vi "GetGlobalDefaultConfiguration.vi"(3 "Read defaults?":bool) -> ()   [LabVIEW 2013]
uses:
  QC_MeasurementSetup.vi
panel:
  out "Configuration File Striptest":path
  out "Configuration File Cis":path
  out "Configuration File Stability":path
  out "Configuration File CV":path
  out "Configuration File IV":path
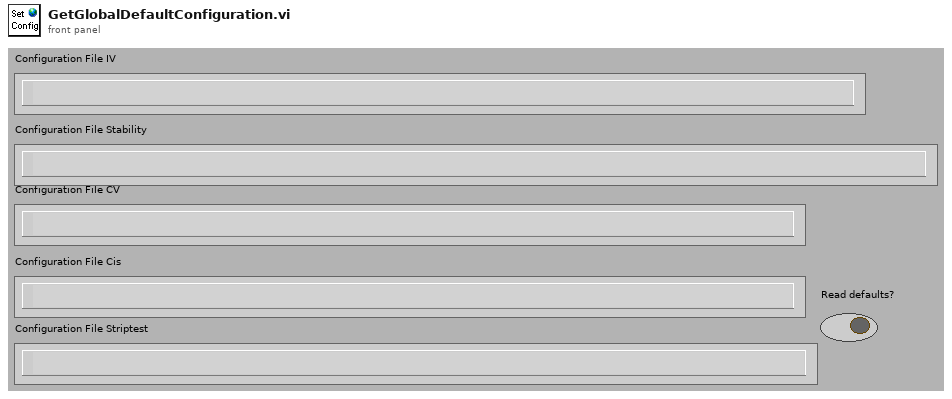
[diagram p1: front panel]
types:
  T1 = cluster{"Supply":refnum<class "SupplyControl.lvclass">, "Arduino":refnum<class "ArduinoControl.lvclass">, "Measurement switch":refnum<class "Switching.lvclass">, "Initial Voltage [V]":dbl, "Final Voltage [V]":dbl, "Step Size [V]":dbl, "Step Interval [s]":i32, "Number Of Steps":u32, "Ramp down steps [V]":dbl, "Ramp down Interval [s]":i32, "hold steps":i32, "Set Current Limit?":bool, "Current Limit [µA]":dbl, "Temperature Readout":enum16{"Read Arduino", "Enter manually"}, "Supply Name":string, "V_breakdown Limit [V]":dbl, "Measurement switch used?":bool}
  T2 = cluster{"Supply":refnum<class "SupplyControl.lvclass">, "LCR":refnum<class "LCRControl.lvclass">, "Arduino":refnum<class "ArduinoControl.lvclass">, "Measurement switch":refnum<class "Switching.lvclass">, "Initial Voltage [V]":dbl, "Final Voltage [V]":dbl, "Step Size [V]":dbl, "Step Interval [s]":i32, "Number Of Steps":u32, "AC frequency [Hz]":i32, "RC Configuration":u16, "AC amplitude [V]":dbl, "Ramp down steps [V]":dbl, "Ramp down Interval [s]":i32, "Set Current Limit?":bool, "Current Limit [µA]":dbl, "Temperature Readout":enum16{"Read Arduino", "Enter manually"}, "Supply Name":string, "LCR Name":string, "V_depletion Limit [V]":dbl, "Measurement switch used?":bool}
  T3 = cluster{"Supply":refnum<class "SupplyControl.lvclass">, "DMM":refnum<class "MultimeterControl.lvclass">, "DUT switch":refnum<class "Switching.lvclass">, "Arduino":refnum<class "ArduinoControl.lvclass">, "Measurement switch":refnum<class "Switching.lvclass">, "Voltage [V]":dbl, "Measurement Interval [s]":i32, "Test Duration":u32, "Ramp up steps [V]":dbl, "Ramp up Interval [s]":u32, "Ramp down steps [V]":dbl, "Ramp down Interval [s]":i32, "Set Current Limit?":bool, "Current Limit [µA]":dbl, "Temperature Readout":enum16{"Read Arduino", "Enter manually"}, "Supply Name":string, "DMM Name":string, "Maximum current fluctuation [%]":dbl, "Measurement switch used?":bool, "DUT switch used?":bool}
  T4 = cluster{"Supply":refnum<class "SupplyControl.lvclass">, "LCR":refnum<class "LCRControl.lvclass">, "Arduino":refnum<class "ArduinoControl.lvclass">, "Measurement switch":refnum<class "Switching.lvclass">, "Initial Voltage [V]":dbl, "Final Voltage [V]":dbl, "Step Size [V]":dbl, "Step Interval [s]":i32, "Number Of Steps":u32, "AC frequency [Hz]":i32, "RC Configuration":u16, "AC amplitude [V]":dbl, "Ramp down steps [V]":dbl, "Ramp down Interval [s]":i32, "Set Current Limit?":bool, "Current Limit [µA]":dbl, "Temperature Readout":enum16{"Read Arduino", "Enter manually"}, "Supply Name":string, "LCR Name":string, "C_is Limit [pF/cm]":dbl, "Measurement switch used?":bool}
  T5 = cluster{"Bias Supply":refnum<class "SupplyControl.lvclass">, "SMU":refnum<class "SupplyControl.lvclass">, "LCR":refnum<class "LCRControl.lvclass">, "ProbeStation":refnum<class "ProbeStationControl.lvclass">, "Arduino":refnum<class "ArduinoControl.lvclass">, "Measurement switch":refnum<class "Switching.lvclass">, "Probe Card Channels":i32, "Bias Voltage [V]":dbl, "First strip":i32, "Last strip":i32, "Base Voltage [V]":dbl, "Base Ramp Step [V]":dbl, "Base Ramp Interval [ms]":u32, "High Voltage [V]":dbl, "High Ramp Step [V]":dbl, "High Ramp Interval [ms]":u32, "AC frequency [Hz]":i32, "AC amplitude [V]":dbl, "RC Configuration":u16, "Single Needle":bool, "Temperature Readout":enum16{"Read Arduino", "Enter manually"}, "Fraction of good strips [%]":dbl, "Measurement switch used?":bool, "Matrix X Channels":cluster{"Mux1 C1":i32, "Mux1 C2":i32, "Mux2 C1":i32, "Mux2 C2":i32}, "Pinholes Y/N":bool, "Capacitance Y/N":bool, "Resistance Y/N":bool, "Bias Supply Name":string, "SMU Name":string, "LCR Name":string}
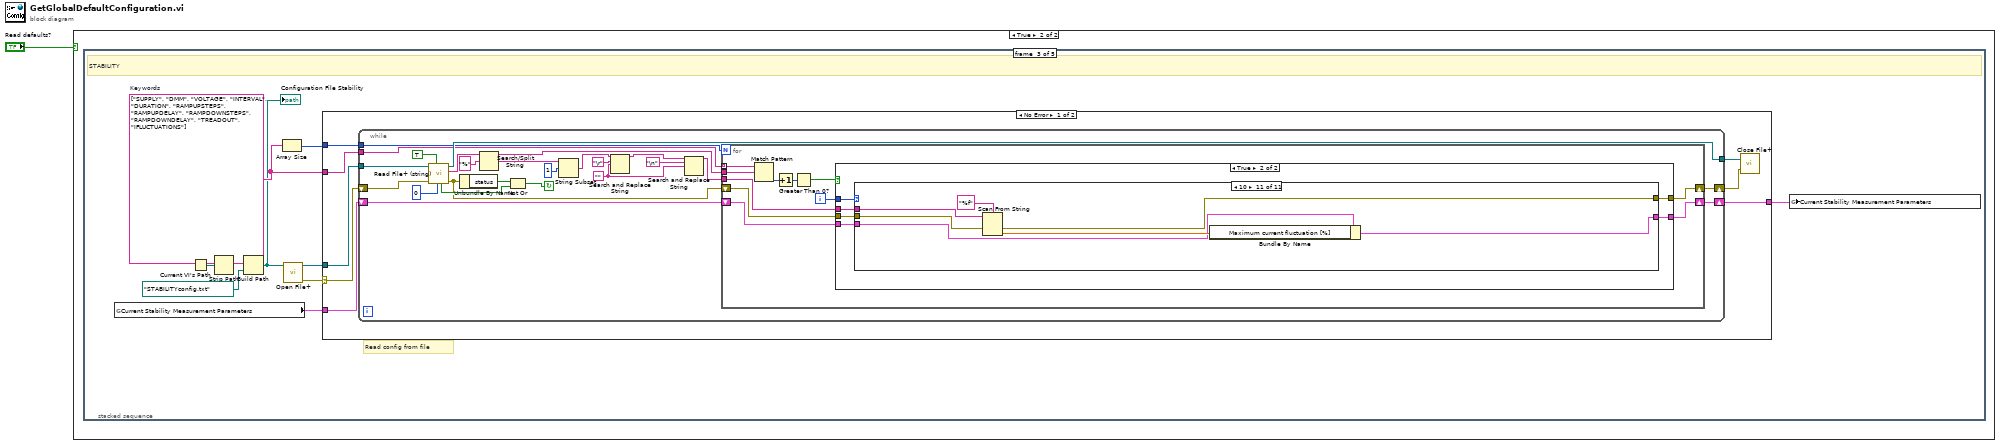
[diagram p0: block diagram]
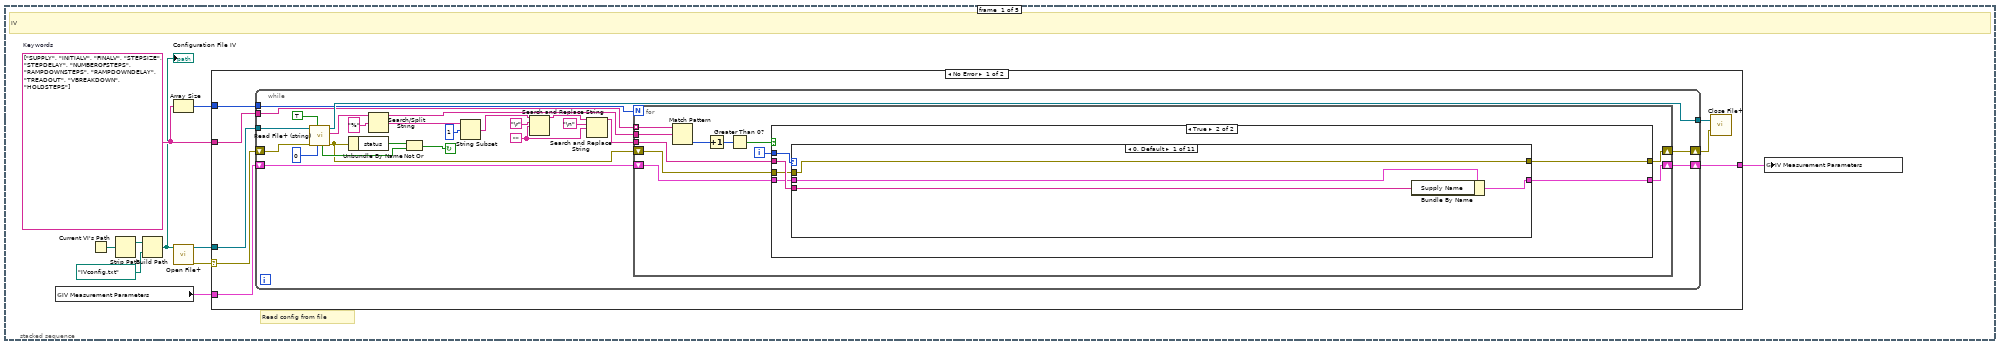
[diagram p3: hidden frame]
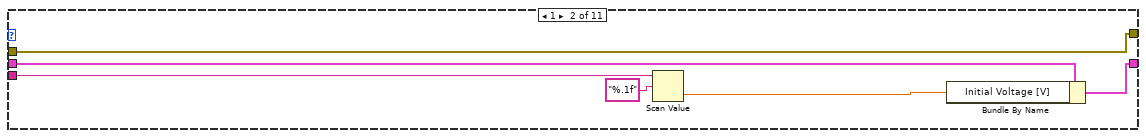
[diagram p5: hidden frame]
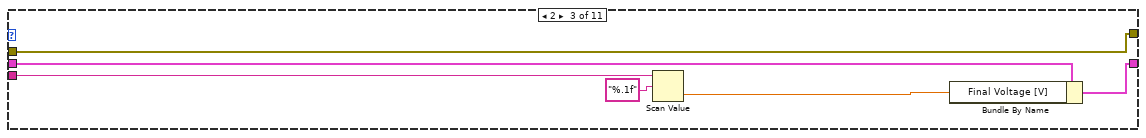
[diagram p6: hidden frame]
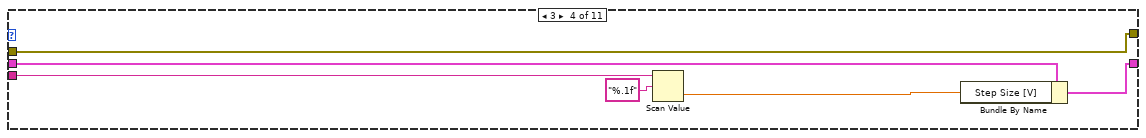
[diagram p7: hidden frame]
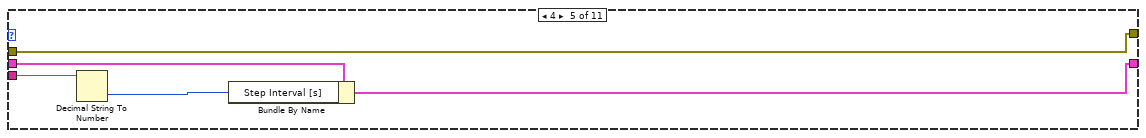
[diagram p8: hidden frame]
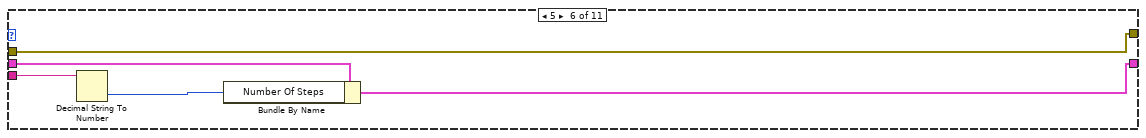
[diagram p9: hidden frame]
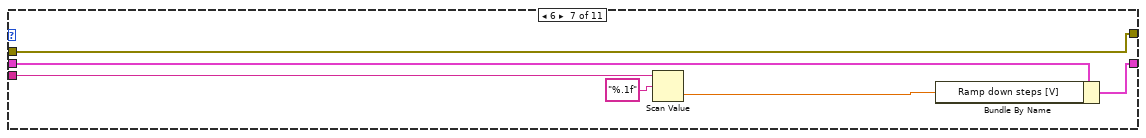
[diagram p10: hidden frame]
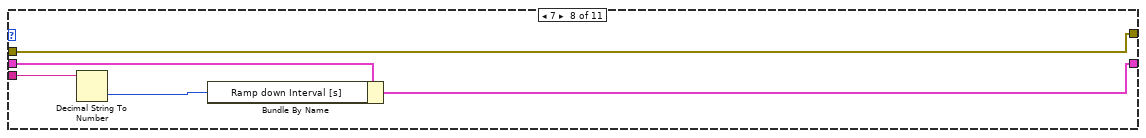
[diagram p11: hidden frame]
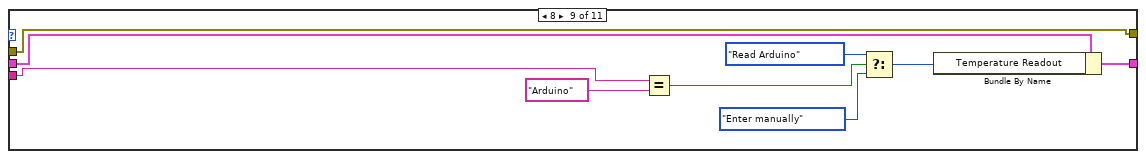
[diagram p12: hidden frame]
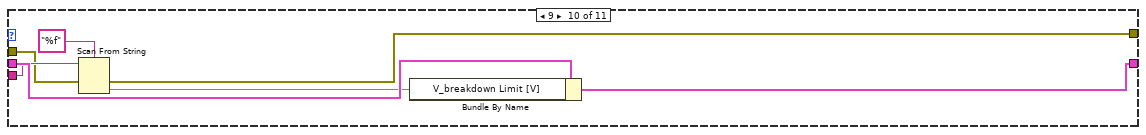
[diagram p13: hidden frame]
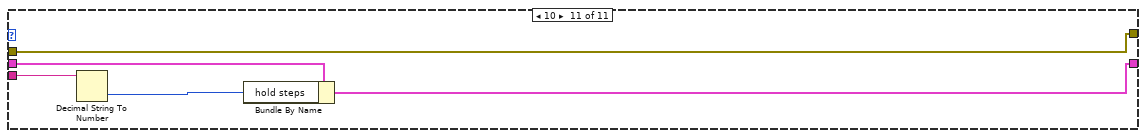
[diagram p14: hidden frame]
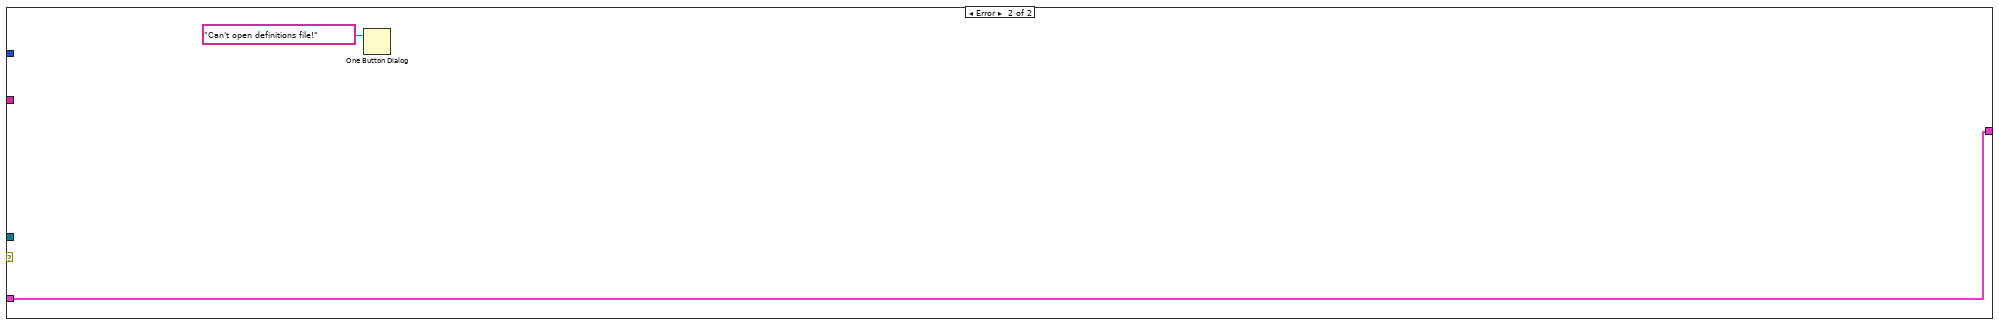
[diagram p15: hidden frame]
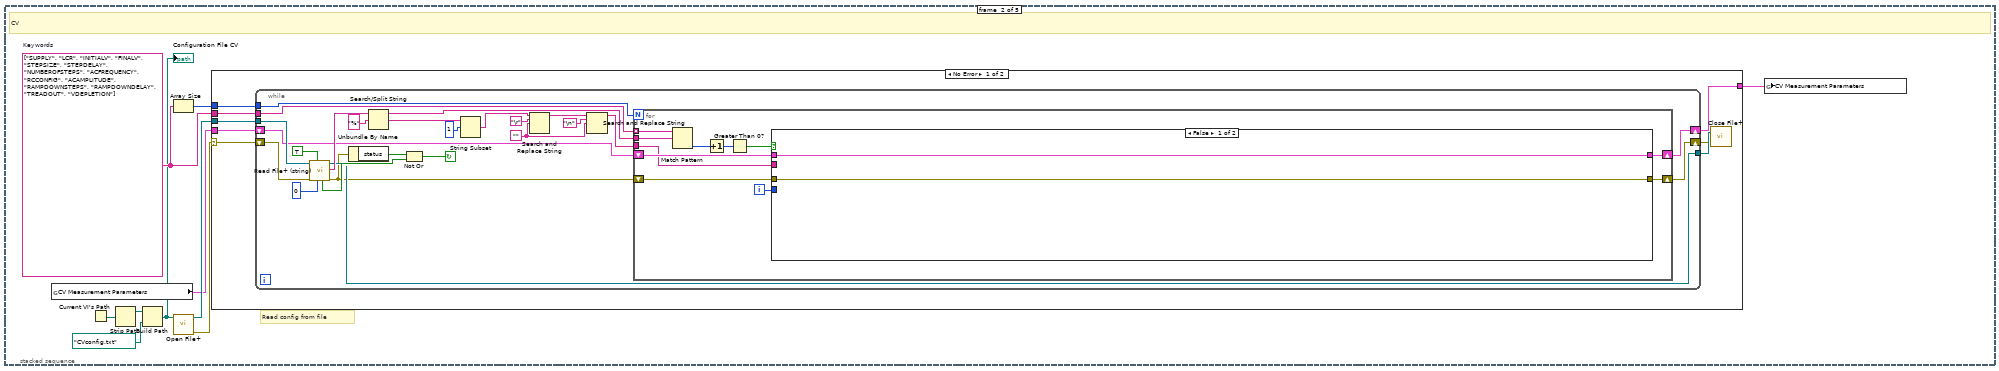
[diagram p16: hidden frame]
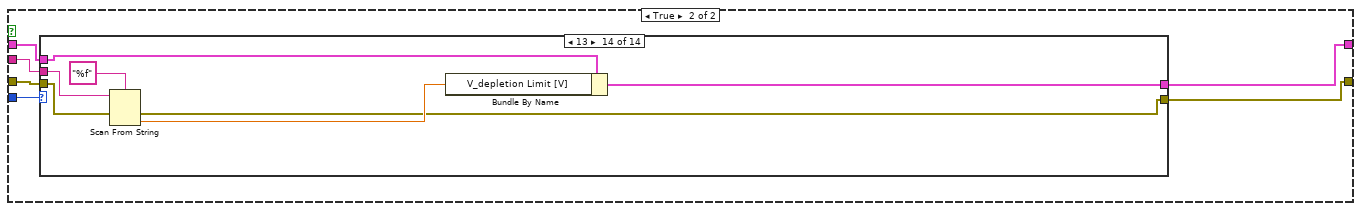
[diagram p17: hidden frame]
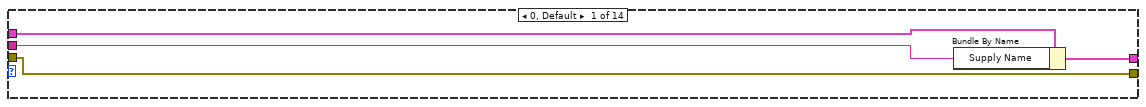
[diagram p18: hidden frame]
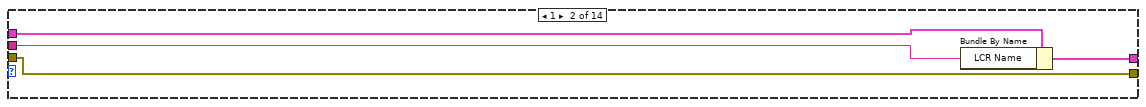
[diagram p19: hidden frame]
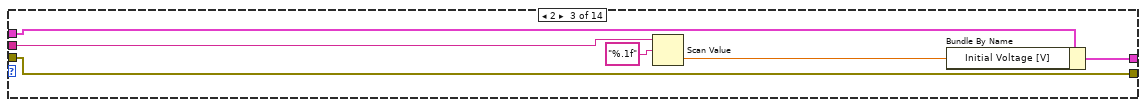
[diagram p20: hidden frame]
diagram:
  n1 = case shown="True" "Read defaults?" {
    frame False {
    }
    frame True {
      n2 = stacked-sequence {
        frame #0 {
          w11 = string[] ["SUPPLY", "INITIALV", "FINALV", "STEPSIZE", "STEPDELAY", "NUMBEROFSTEPS", "RAMPDOWNSTEPS", "RAMPDOWNDELAY", "TREADOUT", "VBREAKDOWN", "HOLDSTEPS"]  # Keywords
          # "Read config from file"
          # "IV"
          n3 = global read "QC_MeasurementSetup.vi" "IV Measurement Parameters"() -> (w2:T1)
          n4 = Current VI's Path() -> (path=w6:path)
          n5 = Strip Path(path=w6) -> (stripped path=w5:path)  [unwired: 1 out]
          n6 = Build Path(base path=w5, name or relative path=path "IVconfig.txt") -> (appended path=w4:path)
          "Configuration File IV" <- w4
          n7 = Array Size(array=w11) -> (size(s)=w10:i32)
          n8 = call <vilib>:"Open File+.vi"("file path (\" \")"=w4) -> ("error out"=w7:errorcluster, "refnum"=w8:refnum<file>)  [unwired: 7 in, 2 out]
          n9 = case shown="No Error" w7 {
            selector: w7 -> [w12 _]
            tunnel: w8 -> [w19 _]
            tunnel: w11 -> [w18 _]
            tunnel: w10 -> [w17 _]
            tunnel: w2 -> [w16 w128]
            tunnel: [w15 w128] -> w3
            frame No Error {
              n10 = while {
                shift-left: w16 -> [w30]
                shift-right: [w29] -> w15
                tunnel: w17 -> [w28]
                tunnel: w18 -> [w32]
                tunnel: [w35] -> w14
                tunnel: w19 -> [w41]
                shift-right: [w26] -> w13
                shift-left: w12 -> [w34]
                stop <- w37 continue-if-true
                w23 = ""
                n11 = call <vilib>:"Read File+ (string).vi"("count"=0, "line mode (characters:F)"=TRUE, "error in (no error)"=w34, "refnum"=w41) -> ("error out"=w27:errorcluster, "string"=w36:string, "dup refnum"=w35:refnum<file>, "EOF?"=w39:bool)  [unwired: 3 in, 1 out]
                n12 = Unbundle By Name(w27) -> ("status"=w38:bool)
                n13 = Search/Split String(string=w36, search string/char (-)="%" ("search char (-)")) -> (substring before match=w31:string, match + rest of string=w42:string)  [unwired: 1 in, 1 out]
                n14 = Not Or(1:w39, 2:w38) -> (0:w37:bool)
                n15 = String Subset(string=w42, offset (0)=1) -> (substring=w21:string)  [unwired: 1 in]
                n16 = Search and Replace String(input string=w21, search string="\r", replace string=w23) -> (result string=w22:string)  [unwired: 5 in, 3 out]
                n17 = Search and Replace String(input string=w22, search string="\n", replace string=w23) -> (result string=w20:string)  [unwired: 5 in, 3 out]
                n18 = for {
                  N: w28 -> [_]
                  tunnel: w32 -> [w53] mode=indexing
                  tunnel: w31 -> [w48]
                  shift-right: [w49] -> w29
                  shift-left: w30 -> [w50]
                  tunnel: w20 -> [w47]
                  shift-right: [w45] -> w26
                  shift-left: w27 -> [w46]
                  i -> [w51]
                  n19 = Match Pattern(string=w53, regular expression=w48) -> (offset past match=w54:i32)  [unwired: 1 in, 3 out]
                  n20 = Increment(x=w54) -> (x+1=w55:i32)
                  n21 = Greater Than 0?(x=w55) -> (x > 0?=w52:bool)
                  n22 = case shown="True" w52 {
                    tunnel: w51 -> [_ w63]
                    tunnel: w47 -> [_ w62]
                    tunnel: w50 -> [w57 w61]
                    tunnel: [w57 w60] -> w49
                    tunnel: w46 -> [w56 w59]
                    tunnel: [w56 w58] -> w45
                    frame False {
                    }
                    frame True {
                      n23 = case shown="0, Default" w63 {
                        tunnel: w62 -> [w65 w71 w76 w82 w88 w93 w98 w104 w113 w120 w124]
                        tunnel: w61 -> [w66 w73 w79 w85 w90 w95 w101 w106 w115 w122 w127]
                        tunnel: [w67 w72 w78 w84 w89 w94 w100 w105 w114 w121 w126] -> w60
                        tunnel: w59 -> [w64 w68 w74 w80 w86 w91 w96 w102 w112 w117 w123]
                        tunnel: [w64 w68 w74 w80 w86 w91 w96 w102 w112 w116 w123] -> w58
                        frame 0, Default {
                          n24 = Bundle By Name(cluster=w66, "Supply Name"=w65) -> (w67:T1)
                        }
                        frame 1 {
                          n25 = Scan Value(string=w71, format string="%.1f") -> (value=w70:dbl)  [unwired: 1 in, 1 out]
                          n26 = Bundle By Name(cluster=w73, "Initial Voltage [V]"=w70) -> (w72:T1)
                        }
                        frame 2 {
                          n27 = Scan Value(string=w76, format string="%.1f") -> (value=w75:dbl)  [unwired: 1 in, 1 out]
                          n28 = Bundle By Name(cluster=w79, "Final Voltage [V]"=w75) -> (w78:T1)
                        }
                        frame 3 {
                          n29 = Scan Value(string=w82, format string="%.1f") -> (value=w81:dbl)  [unwired: 1 in, 1 out]
                          n30 = Bundle By Name(cluster=w85, "Step Size [V]"=w81) -> (w84:T1)
                        }
                        frame 4 {
                          n31 = Decimal String To Number(string=w88) -> (number=w87:i32)  [unwired: 2 in, 1 out]
                          n32 = Bundle By Name(cluster=w90, "Step Interval [s]"=w87) -> (w89:T1)
                        }
                        frame 5 {
                          n33 = Decimal String To Number(string=w93) -> (number=w92:i32)  [unwired: 2 in, 1 out]
                          n34 = Bundle By Name(cluster=w95, "Number Of Steps"=w92) -> (w94:T1)
                        }
                        frame 6 {
                          n35 = Scan Value(string=w98, format string="%.1f") -> (value=w97:dbl)  [unwired: 1 in, 1 out]
                          n36 = Bundle By Name(cluster=w101, "Ramp down steps [V]"=w97) -> (w100:T1)
                        }
                        frame 7 {
                          n37 = Decimal String To Number(string=w104) -> (number=w103:i32)  [unwired: 2 in, 1 out]
                          n38 = Bundle By Name(cluster=w106, "Ramp down Interval [s]"=w103) -> (w105:T1)
                        }
                        frame 8 {
                          n39 = Equal?(x=w113, y="Arduino") -> (x = y?=w110:bool)
                          n40 = Select(t=enum16{"Read Arduino", "Enter manually"}."Read Arduino" ("Temperature Readout"), s=w110, f=enum16{"Read Arduino", "Enter manually"}."Enter manually" ("Temperature Readout")) -> (s? t:f=w107:enum16{"Read Arduino", "Enter manually"})
                          n41 = Bundle By Name(cluster=w115, "Temperature Readout"=w107) -> (w114:T1)
                        }
                        frame 9 {
                          n42 = Scan From String(format string="%f", input string=w120, error in=w117) -> (error out=w116:errorcluster, output 1=w119:dbl)  [unwired: 2 in, 2 out]
                          n43 = Bundle By Name(cluster=w122, "V_breakdown Limit [V]"=w119) -> (w121:T1)
                        }
                        frame 10 {
                          n44 = Decimal String To Number(string=w124) -> (number=w125:i32)  [unwired: 2 in, 1 out]
                          n45 = Bundle By Name(cluster=w127, "hold steps"=w125) -> (w126:T1)
                        }
                      }
                    }
                  }
                }
              }
              n46 = call <vilib>:"Close File+.vi"("error in (no error)"=w13, "refnum"=w14) -> ()  [unwired: 3 in, 3 out]
            }
            frame Error {
              n47 = One Button Dialog(message="Can't open definitions file!") -> ()  [unwired: 1 in, 1 out]
            }
          }
          n48 = global write "QC_MeasurementSetup.vi" "IV Measurement Parameters"(w3) -> ()
        }
        frame #1 {
          w139 = string[] ["SUPPLY", "LCR", "INITIALV", "FINALV", "STEPSIZE", "STEPDELAY", "NUMBEROFSTEPS", "ACFREQUENCY", "RCCONFIG", "ACAMPLITUDE", "RAMPDOWNSTEPS", "RAMPDOWNDELAY", "TREADOUT", "VDEPLETION"]  # Keywords
          # "Read config from file"
          # "CV"
          n49 = global read "QC_MeasurementSetup.vi" "CV Measurement Parameters"() -> (w130:T2)
          n50 = Current VI's Path() -> (path=w134:path)
          n51 = Strip Path(path=w134) -> (stripped path=w133:path)  [unwired: 1 out]
          n52 = Build Path(base path=w133, name or relative path=path "CVconfig.txt") -> (appended path=w132:path)
          "Configuration File CV" <- w132
          n53 = Array Size(array=w139) -> (size(s)=w138:i32)
          n54 = call <vilib>:"Open File+.vi"("file path (\" \")"=w132) -> ("error out"=w135:errorcluster, "refnum"=w136:refnum<file>)  [unwired: 7 in, 2 out]
          n55 = case shown="No Error" w135 {
            selector: w135 -> [w140 _]
            tunnel: w136 -> [w147 _]
            tunnel: w139 -> [w146 _]
            tunnel: w138 -> [w145 _]
            tunnel: w130 -> [w144 w275]
            tunnel: [w143 w275] -> w131
            frame No Error {
              n56 = while {
                shift-left: w144 -> [w158]
                shift-right: [w157] -> w143
                tunnel: w145 -> [w156]
                tunnel: w146 -> [w160]
                tunnel: [w163] -> w142
                tunnel: w147 -> [w169]
                shift-right: [w154] -> w141
                shift-left: w140 -> [w162]
                stop <- w165 continue-if-true
                w151 = ""
                n57 = call <vilib>:"Read File+ (string).vi"("count"=0, "line mode (characters:F)"=TRUE, "error in (no error)"=w162, "refnum"=w169) -> ("error out"=w155:errorcluster, "string"=w164:string, "dup refnum"=w163:refnum<file>, "EOF?"=w167:bool)  [unwired: 3 in, 1 out]
                n58 = Unbundle By Name(w155) -> ("status"=w166:bool)
                n59 = Search/Split String(string=w164, search string/char (-)="%" ("search char (-)")) -> (substring before match=w159:string, match + rest of string=w170:string)  [unwired: 1 in, 1 out]
                n60 = Not Or(1:w167, 2:w166) -> (0:w165:bool)
                n61 = String Subset(string=w170, offset (0)=1) -> (substring=w149:string)  [unwired: 1 in]
                n62 = Search and Replace String(input string=w149, search string="\r", replace string=w151) -> (result string=w150:string)  [unwired: 5 in, 3 out]
                n63 = Search and Replace String(input string=w150, search string="\n", replace string=w151) -> (result string=w148:string)  [unwired: 5 in, 3 out]
                n64 = for {
                  N: w156 -> [_]
                  tunnel: w160 -> [w181] mode=indexing
                  tunnel: w159 -> [w176]
                  shift-right: [w177] -> w157
                  shift-left: w158 -> [w178]
                  tunnel: w148 -> [w175]
                  shift-right: [w173] -> w154
                  shift-left: w155 -> [w174]
                  i -> [w179]
                  n65 = Match Pattern(string=w181, regular expression=w176) -> (offset past match=w182:i32)  [unwired: 1 in, 3 out]
                  n66 = Increment(x=w182) -> (x+1=w183:i32)
                  n67 = Greater Than 0?(x=w183) -> (x > 0?=w180:bool)
                  n68 = case shown="False" w180 {
                    tunnel: w179 -> [_ w191]
                    tunnel: w175 -> [_ w190]
                    tunnel: w178 -> [w185 w189]
                    tunnel: [w185 w188] -> w177
                    tunnel: w174 -> [w184 w187]
                    tunnel: [w184 w186] -> w173
                    frame False {
                    }
                    frame True {
                      n69 = case shown="13" w191 {
                        tunnel: w190 -> [w193 w197 w203 w208 w214 w220 w225 w230 w238 w247 w250 w256 w265 w272]
                        tunnel: w189 -> [w194 w198 w205 w211 w217 w222 w227 w232 w241 w245 w253 w258 w267 w268]
                        tunnel: [w195 w199 w204 w210 w216 w221 w226 w231 w240 w243 w252 w257 w266 w269] -> w188
                        tunnel: w187 -> [w192 w196 w200 w206 w212 w218 w223 w228 w233 w242 w248 w254 w264 w271]
                        tunnel: [w192 w196 w200 w206 w212 w218 w223 w228 w233 w242 w248 w254 w264 w270] -> w186
                        frame 0, Default {
                          n70 = Bundle By Name(cluster=w194, "Supply Name"=w193) -> (w195:T2)
                        }
                        frame 1 {
                          n71 = Bundle By Name(cluster=w198, "LCR Name"=w197) -> (w199:T2)
                        }
                        frame 2 {
                          n72 = Scan Value(string=w203, format string="%.1f") -> (value=w202:dbl)  [unwired: 1 in, 1 out]
                          n73 = Bundle By Name(cluster=w205, "Initial Voltage [V]"=w202) -> (w204:T2)
                        }
                        frame 3 {
                          n74 = Scan Value(string=w208, format string="%.1f") -> (value=w207:dbl)  [unwired: 1 in, 1 out]
                          n75 = Bundle By Name(cluster=w211, "Final Voltage [V]"=w207) -> (w210:T2)
                        }
                        frame 4 {
                          n76 = Scan Value(string=w214, format string="%.1f") -> (value=w213:dbl)  [unwired: 1 in, 1 out]
                          n77 = Bundle By Name(cluster=w217, "Step Size [V]"=w213) -> (w216:T2)
                        }
                        frame 5 {
                          n78 = Decimal String To Number(string=w220) -> (number=w219:i32)  [unwired: 2 in, 1 out]
                          n79 = Bundle By Name(cluster=w222, "Step Interval [s]"=w219) -> (w221:T2)
                        }
                        frame 6 {
                          n80 = Decimal String To Number(string=w225) -> (number=w224:i32)  [unwired: 2 in, 1 out]
                          n81 = Bundle By Name(cluster=w227, "Number Of Steps"=w224) -> (w226:T2)
                        }
                        frame 7 {
                          n82 = Decimal String To Number(string=w230) -> (number=w229:i32)  [unwired: 2 in, 1 out]
                          n83 = Bundle By Name(cluster=w232, "AC frequency [Hz]"=w229) -> (w231:T2)
                        }
                        frame 8 {
                          w237 = u16 0 items=["serial", "parallel"] ("RC Configuration")
                          w236 = u16 1 items=["serial", "parallel"] ("RC Configuration")
                          n84 = Equal?(x=w238, y="serial") -> (x = y?=w235:bool)
                          n85 = Select(t=w237, s=w235, f=w236) -> (s? t:f=w234:u16)
                          n86 = Bundle By Name(cluster=w241, "RC Configuration"=w234) -> (w240:T2)
                        }
                        frame 9 {
                          n87 = Scan Value(string=w247, format string="%.1f") -> (value=w244:dbl)  [unwired: 1 in, 1 out]
                          n88 = Bundle By Name(cluster=w245, "AC amplitude [V]"=w244) -> (w243:T2)
                        }
                        frame 10 {
                          n89 = Scan Value(string=w250, format string="%.1f") -> (value=w249:dbl)  [unwired: 1 in, 1 out]
                          n90 = Bundle By Name(cluster=w253, "Ramp down steps [V]"=w249) -> (w252:T2)
                        }
                        frame 11 {
                          n91 = Decimal String To Number(string=w256) -> (number=w255:i32)  [unwired: 2 in, 1 out]
                          n92 = Bundle By Name(cluster=w258, "Ramp down Interval [s]"=w255) -> (w257:T2)
                        }
                        frame 12 {
                          n93 = Equal?(x=w265, y="Arduino") -> (x = y?=w262:bool)
                          n94 = Select(t=enum16{"Read Arduino", "Enter manually"}."Read Arduino" ("Temperature Readout"), s=w262, f=enum16{"Read Arduino", "Enter manually"}."Enter manually" ("Temperature Readout")) -> (s? t:f=w259:enum16{"Read Arduino", "Enter manually"})
                          n95 = Bundle By Name(cluster=w267, "Temperature Readout"=w259) -> (w266:T2)
                        }
                        frame 13 {
                          n96 = Scan From String(format string="%f", input string=w272, error in=w271) -> (error out=w270:errorcluster, output 1=w274:dbl)  [unwired: 2 in, 2 out]
                          n97 = Bundle By Name(cluster=w268, "V_depletion Limit [V]"=w274) -> (w269:T2)
                        }
                      }
                    }
                  }
                }
              }
              n98 = call <vilib>:"Close File+.vi"("error in (no error)"=w141, "refnum"=w142) -> ()  [unwired: 3 in, 3 out]
            }
            frame Error {
              n99 = One Button Dialog(message="Can't open definitions file!") -> ()  [unwired: 1 in, 1 out]
            }
          }
          n100 = global write "QC_MeasurementSetup.vi" "CV Measurement Parameters"(w131) -> ()
        }
        frame #2 {
          w286 = string[] ["SUPPLY", "DMM", "VOLTAGE", "INTERVAL", "DURATION", "RAMPUPSTEPS", "RAMPUPDELAY", "RAMPDOWNSTEPS", "RAMPDOWNDELAY", "TREADOUT", "IFLUCTUATIONS"]  # Keywords
          # "Read config from file"
          # "STABILITY"
          n101 = global read "QC_MeasurementSetup.vi" "Current Stability Measurement Parameters"() -> (w277:T3)
          n102 = Current VI's Path() -> (path=w281:path)
          n103 = Strip Path(path=w281) -> (stripped path=w280:path)  [unwired: 1 out]
          n104 = Build Path(base path=w280, name or relative path=path "STABILITYconfig.txt") -> (appended path=w279:path)
          "Configuration File Stability" <- w279
          n105 = Array Size(array=w286) -> (size(s)=w285:i32)
          n106 = call <vilib>:"Open File+.vi"("file path (\" \")"=w279) -> ("error out"=w282:errorcluster, "refnum"=w283:refnum<file>)  [unwired: 7 in, 2 out]
          n107 = case shown="No Error" w282 {
            selector: w282 -> [w287 _]
            tunnel: w283 -> [w294 _]
            tunnel: w286 -> [w293 _]
            tunnel: w285 -> [w292 _]
            tunnel: w277 -> [w291 w401]
            tunnel: [w290 w401] -> w278
            frame No Error {
              n108 = while {
                shift-left: w291 -> [w305]
                shift-right: [w304] -> w290
                tunnel: w292 -> [w303]
                tunnel: w293 -> [w307]
                tunnel: [w310] -> w289
                tunnel: w294 -> [w316]
                shift-right: [w301] -> w288
                shift-left: w287 -> [w309]
                stop <- w312 continue-if-true
                w298 = ""
                n109 = call <vilib>:"Read File+ (string).vi"("count"=0, "line mode (characters:F)"=TRUE, "error in (no error)"=w309, "refnum"=w316) -> ("error out"=w302:errorcluster, "string"=w311:string, "dup refnum"=w310:refnum<file>, "EOF?"=w314:bool)  [unwired: 3 in, 1 out]
                n110 = Unbundle By Name(w302) -> ("status"=w313:bool)
                n111 = Search/Split String(string=w311, search string/char (-)="%" ("search char (-)")) -> (substring before match=w306:string, match + rest of string=w317:string)  [unwired: 1 in, 1 out]
                n112 = Not Or(1:w314, 2:w313) -> (0:w312:bool)
                n113 = String Subset(string=w317, offset (0)=1) -> (substring=w296:string)  [unwired: 1 in]
                n114 = Search and Replace String(input string=w296, search string="\r", replace string=w298) -> (result string=w297:string)  [unwired: 5 in, 3 out]
                n115 = Search and Replace String(input string=w297, search string="\n", replace string=w298) -> (result string=w295:string)  [unwired: 5 in, 3 out]
                n116 = for {
                  N: w303 -> [_]
                  tunnel: w307 -> [w328] mode=indexing
                  tunnel: w306 -> [w323]
                  shift-right: [w324] -> w304
                  shift-left: w305 -> [w325]
                  tunnel: w295 -> [w322]
                  shift-right: [w320] -> w301
                  shift-left: w302 -> [w321]
                  i -> [w326]
                  n117 = Match Pattern(string=w328, regular expression=w323) -> (offset past match=w329:i32)  [unwired: 1 in, 3 out]
                  n118 = Increment(x=w329) -> (x+1=w330:i32)
                  n119 = Greater Than 0?(x=w330) -> (x > 0?=w327:bool)
                  n120 = case shown="True" w327 {
                    tunnel: w326 -> [_ w338]
                    tunnel: w322 -> [_ w337]
                    tunnel: w325 -> [w332 w336]
                    tunnel: [w332 w335] -> w324
                    tunnel: w321 -> [w331 w334]
                    tunnel: [w331 w333] -> w320
                    frame False {
                    }
                    frame True {
                      n121 = case shown="10" w338 {
                        tunnel: w337 -> [w339 w343 w350 w354 w359 w365 w371 w376 w382 w391 w397]
                        tunnel: w336 -> [w341 w345 w352 w357 w362 w368 w373 w379 w384 w393 w398]
                        tunnel: [w342 w346 w351 w356 w361 w367 w372 w378 w383 w392 w396] -> w335
                        tunnel: w334 -> [w340 w344 w347 w355 w360 w366 w369 w374 w380 w390 w394]
                        tunnel: [w340 w344 w347 w355 w360 w366 w369 w374 w380 w390 w395] -> w333
                        frame 0, Default {
                          n122 = Bundle By Name(cluster=w341, "Supply Name"=w339) -> (w342:T3)
                        }
                        frame 1 {
                          n123 = Bundle By Name(cluster=w345, "DMM Name"=w343) -> (w346:T3)
                        }
                        frame 2 {
                          n124 = Scan Value(string=w350, format string="%.1f") -> (value=w349:dbl)  [unwired: 1 in, 1 out]
                          n125 = Bundle By Name(cluster=w352, "Voltage [V]"=w349) -> (w351:T3)
                        }
                        frame 3 {
                          n126 = Decimal String To Number(string=w354) -> (number=w353:i32)  [unwired: 2 in, 1 out]
                          n127 = Bundle By Name(cluster=w357, "Measurement Interval [s]"=w353) -> (w356:T3)
                        }
                        frame 4 {
                          n128 = Decimal String To Number(string=w359) -> (number=w358:i32)  [unwired: 2 in, 1 out]
                          n129 = Bundle By Name(cluster=w362, "Test Duration"=w358) -> (w361:T3)
                        }
                        frame 5 {
                          n130 = Scan Value(string=w365, format string="%.1f") -> (value=w363:dbl)  [unwired: 1 in, 1 out]
                          n131 = Bundle By Name(cluster=w368, "Ramp up steps [V]"=w363) -> (w367:T3)
                        }
                        frame 6 {
                          n132 = Decimal String To Number(string=w371) -> (number=w370:i32)  [unwired: 2 in, 1 out]
                          n133 = Bundle By Name(cluster=w373, "Ramp up Interval [s]"=w370) -> (w372:T3)
                        }
                        frame 7 {
                          n134 = Scan Value(string=w376, format string="%.1f") -> (value=w375:dbl)  [unwired: 1 in, 1 out]
                          n135 = Bundle By Name(cluster=w379, "Ramp down steps [V]"=w375) -> (w378:T3)
                        }
                        frame 8 {
                          n136 = Decimal String To Number(string=w382) -> (number=w381:i32)  [unwired: 2 in, 1 out]
                          n137 = Bundle By Name(cluster=w384, "Ramp down Interval [s]"=w381) -> (w383:T3)
                        }
                        frame 9 {
                          n138 = Equal?(x=w391, y="Arduino") -> (x = y?=w388:bool)
                          n139 = Select(t=enum16{"Read Arduino", "Enter manually"}."Read Arduino" ("Temperature Readout"), s=w388, f=enum16{"Read Arduino", "Enter manually"}."Enter manually" ("Temperature Readout")) -> (s? t:f=w385:enum16{"Read Arduino", "Enter manually"})
                          n140 = Bundle By Name(cluster=w393, "Temperature Readout"=w385) -> (w392:T3)
                        }
                        frame 10 {
                          n141 = Scan From String(format string="%f", input string=w397, error in=w394) -> (error out=w395:errorcluster, output 1=w400:dbl)  [unwired: 2 in, 2 out]
                          n142 = Bundle By Name(cluster=w398, "Maximum current fluctuation [%]"=w400) -> (w396:T3)
                        }
                      }
                    }
                  }
                }
              }
              n143 = call <vilib>:"Close File+.vi"("error in (no error)"=w288, "refnum"=w289) -> ()  [unwired: 3 in, 3 out]
            }
            frame Error {
              n144 = One Button Dialog(message="Can't open definitions file!") -> ()  [unwired: 1 in, 1 out]
            }
          }
          n145 = global write "QC_MeasurementSetup.vi" "Current Stability Measurement Parameters"(w278) -> ()
        }
        frame #3 {
          w412 = string[] ["SUPPLY", "LCR", "INITIALV", "FINALV", "STEPSIZE", "STEPDELAY", "NUMBEROFSTEPS", "ACFREQUENCY", "RCCONFIG", "ACAMPLITUDE", "RAMPDOWNSTEPS", "RAMPDOWNDELAY", "TREADOUT", "CISLIMIT"]  # Keywords
          # "Read config from file"
          # "CIS"
          n146 = global read "QC_MeasurementSetup.vi" "Cis Measurement Parameters"() -> (w403:T4)
          n147 = Current VI's Path() -> (path=w407:path)
          n148 = Strip Path(path=w407) -> (stripped path=w406:path)  [unwired: 1 out]
          n149 = Build Path(base path=w406, name or relative path=path "CISconfig.txt") -> (appended path=w405:path)
          "Configuration File Cis" <- w405
          n150 = Array Size(array=w412) -> (size(s)=w411:i32)
          n151 = call <vilib>:"Open File+.vi"("file path (\" \")"=w405) -> ("error out"=w408:errorcluster, "refnum"=w409:refnum<file>)  [unwired: 7 in, 2 out]
          n152 = case shown="No Error" w408 {
            selector: w408 -> [w413 _]
            tunnel: w409 -> [w420 _]
            tunnel: w412 -> [w419 _]
            tunnel: w411 -> [w418 _]
            tunnel: w403 -> [w417 w548]
            tunnel: [w416 w548] -> w404
            frame No Error {
              n153 = while {
                shift-left: w417 -> [w431]
                shift-right: [w430] -> w416
                tunnel: w418 -> [w429]
                tunnel: w419 -> [w433]
                tunnel: [w436] -> w415
                tunnel: w420 -> [w442]
                shift-right: [w427] -> w414
                shift-left: w413 -> [w435]
                stop <- w438 continue-if-true
                w424 = ""
                n154 = call <vilib>:"Read File+ (string).vi"("count"=0, "line mode (characters:F)"=TRUE, "error in (no error)"=w435, "refnum"=w442) -> ("error out"=w428:errorcluster, "string"=w437:string, "dup refnum"=w436:refnum<file>, "EOF?"=w440:bool)  [unwired: 3 in, 1 out]
                n155 = Unbundle By Name(w428) -> ("status"=w439:bool)
                n156 = Search/Split String(string=w437, search string/char (-)="%" ("search char (-)")) -> (substring before match=w432:string, match + rest of string=w443:string)  [unwired: 1 in, 1 out]
                n157 = Not Or(1:w440, 2:w439) -> (0:w438:bool)
                n158 = String Subset(string=w443, offset (0)=1) -> (substring=w422:string)  [unwired: 1 in]
                n159 = Search and Replace String(input string=w422, search string="\r", replace string=w424) -> (result string=w423:string)  [unwired: 5 in, 3 out]
                n160 = Search and Replace String(input string=w423, search string="\n", replace string=w424) -> (result string=w421:string)  [unwired: 5 in, 3 out]
                n161 = for {
                  N: w429 -> [_]
                  tunnel: w433 -> [w454] mode=indexing
                  tunnel: w432 -> [w449]
                  shift-right: [w450] -> w430
                  shift-left: w431 -> [w451]
                  tunnel: w421 -> [w448]
                  shift-right: [w446] -> w427
                  shift-left: w428 -> [w447]
                  i -> [w452]
                  n162 = Match Pattern(string=w454, regular expression=w449) -> (offset past match=w455:i32)  [unwired: 1 in, 3 out]
                  n163 = Increment(x=w455) -> (x+1=w456:i32)
                  n164 = Greater Than 0?(x=w456) -> (x > 0?=w453:bool)
                  n165 = case shown="True" w453 {
                    tunnel: w452 -> [_ w464]
                    tunnel: w448 -> [_ w463]
                    tunnel: w451 -> [w458 w462]
                    tunnel: [w458 w461] -> w450
                    tunnel: w447 -> [w457 w460]
                    tunnel: [w457 w459] -> w446
                    frame False {
                    }
                    frame True {
                      n166 = case shown="0, Default" w464 {
                        tunnel: w463 -> [w465 w469 w476 w481 w487 w493 w498 w503 w511 w520 w523 w529 w538 w545]
                        tunnel: w462 -> [w467 w471 w478 w484 w490 w495 w500 w505 w514 w518 w526 w531 w540 w544]
                        tunnel: [w468 w472 w477 w483 w489 w494 w499 w504 w513 w516 w525 w530 w539 w543] -> w461
                        tunnel: w460 -> [w466 w470 w473 w479 w485 w491 w496 w501 w506 w515 w521 w527 w537 w541]
                        tunnel: [w466 w470 w473 w479 w485 w491 w496 w501 w506 w515 w521 w527 w537 w542] -> w459
                        frame 0, Default {
                          n167 = Bundle By Name(cluster=w467, "Supply Name"=w465) -> (w468:T4)
                        }
                        frame 1 {
                          n168 = Bundle By Name(cluster=w471, "LCR Name"=w469) -> (w472:T4)
                        }
                        frame 2 {
                          n169 = Scan Value(string=w476, format string="%.1f") -> (value=w475:dbl)  [unwired: 1 in, 1 out]
                          n170 = Bundle By Name(cluster=w478, "Initial Voltage [V]"=w475) -> (w477:T4)
                        }
                        frame 3 {
                          n171 = Scan Value(string=w481, format string="%.1f") -> (value=w480:dbl)  [unwired: 1 in, 1 out]
                          n172 = Bundle By Name(cluster=w484, "Final Voltage [V]"=w480) -> (w483:T4)
                        }
                        frame 4 {
                          n173 = Scan Value(string=w487, format string="%.1f") -> (value=w486:dbl)  [unwired: 1 in, 1 out]
                          n174 = Bundle By Name(cluster=w490, "Step Size [V]"=w486) -> (w489:T4)
                        }
                        frame 5 {
                          n175 = Decimal String To Number(string=w493) -> (number=w492:i32)  [unwired: 2 in, 1 out]
                          n176 = Bundle By Name(cluster=w495, "Step Interval [s]"=w492) -> (w494:T4)
                        }
                        frame 6 {
                          n177 = Decimal String To Number(string=w498) -> (number=w497:i32)  [unwired: 2 in, 1 out]
                          n178 = Bundle By Name(cluster=w500, "Number Of Steps"=w497) -> (w499:T4)
                        }
                        frame 7 {
                          n179 = Decimal String To Number(string=w503) -> (number=w502:i32)  [unwired: 2 in, 1 out]
                          n180 = Bundle By Name(cluster=w505, "AC frequency [Hz]"=w502) -> (w504:T4)
                        }
                        frame 8 {
                          w510 = u16 0 items=["serial", "parallel"] ("RC Configuration")
                          w509 = u16 1 items=["serial", "parallel"] ("RC Configuration")
                          n181 = Equal?(x=w511, y="serial") -> (x = y?=w508:bool)
                          n182 = Select(t=w510, s=w508, f=w509) -> (s? t:f=w507:u16)
                          n183 = Bundle By Name(cluster=w514, "RC Configuration"=w507) -> (w513:T4)
                        }
                        frame 9 {
                          n184 = Scan Value(string=w520, format string="%.1f") -> (value=w517:dbl)  [unwired: 1 in, 1 out]
                          n185 = Bundle By Name(cluster=w518, "AC amplitude [V]"=w517) -> (w516:T4)
                        }
                        frame 10 {
                          n186 = Scan Value(string=w523, format string="%.1f") -> (value=w522:dbl)  [unwired: 1 in, 1 out]
                          n187 = Bundle By Name(cluster=w526, "Ramp down steps [V]"=w522) -> (w525:T4)
                        }
                        frame 11 {
                          n188 = Decimal String To Number(string=w529) -> (number=w528:i32)  [unwired: 2 in, 1 out]
                          n189 = Bundle By Name(cluster=w531, "Ramp down Interval [s]"=w528) -> (w530:T4)
                        }
                        frame 12 {
                          n190 = Equal?(x=w538, y="Arduino") -> (x = y?=w535:bool)
                          n191 = Select(t=enum16{"Read Arduino", "Enter manually"}."Read Arduino" ("Temperature Readout"), s=w535, f=enum16{"Read Arduino", "Enter manually"}."Enter manually" ("Temperature Readout")) -> (s? t:f=w532:enum16{"Read Arduino", "Enter manually"})
                          n192 = Bundle By Name(cluster=w540, "Temperature Readout"=w532) -> (w539:T4)
                        }
                        frame 13 {
                          n193 = Scan From String(format string="%f", input string=w545, error in=w541) -> (error out=w542:errorcluster, output 1=w547:dbl)  [unwired: 2 in, 2 out]
                          n194 = Bundle By Name(cluster=w544, "C_is Limit [pF/cm]"=w547) -> (w543:T4)
                        }
                      }
                    }
                  }
                }
              }
              n195 = call <vilib>:"Close File+.vi"("error in (no error)"=w414, "refnum"=w415) -> ()  [unwired: 3 in, 3 out]
            }
            frame Error {
              n196 = One Button Dialog(message="Can't open definitions file!") -> ()  [unwired: 1 in, 1 out]
            }
          }
          n197 = global write "QC_MeasurementSetup.vi" "Cis Measurement Parameters"(w404) -> ()
        }
        frame #4 {
          w559 = string[] ["BIASSUPPLY", "SMU", "LCR", "BIASV", "BASEV", "BASERAMP", "BASEINT", "HIGHV", "HIGHRAMP", "HIGHINT", "ACFREQUENCY", "RCCONFIG", "ACAMPLITUDE", "TREADOUT", "GOODSTRIPS", "CARD"]  # Keywords
          # "Read config from file"
          # "STRIPTEST"
          n198 = global read "QC_MeasurementSetup.vi" "Striptest Measurement Parameters"() -> (w551:T5)
          n199 = Current VI's Path() -> (path=w554:path)
          n200 = Strip Path(path=w554) -> (stripped path=w553:path)  [unwired: 1 out]
          n201 = Build Path(base path=w553, name or relative path=path "STRIPTESTconfig.txt") -> (appended path=w550:path)
          "Configuration File Striptest" <- w550
          n202 = Array Size(array=w559) -> (size(s)=w558:i32)
          n203 = call <vilib>:"Open File+.vi"("file path (\" \")"=w550) -> ("error out"=w555:errorcluster, "refnum"=w556:refnum<file>)  [unwired: 7 in, 2 out]
          n204 = case shown="No Error" w555 {
            selector: w555 -> [w560 _]
            tunnel: w556 -> [w567 _]
            tunnel: w559 -> [w566 _]
            tunnel: w558 -> [w565 _]
            tunnel: w551 -> [w564 w704]
            tunnel: [w563 w704] -> w552
            frame No Error {
              n205 = while {
                shift-left: w564 -> [w578]
                shift-right: [w577] -> w563
                tunnel: w565 -> [w576]
                tunnel: w566 -> [w580]
                tunnel: [w583] -> w562
                tunnel: w567 -> [w589]
                shift-right: [w574] -> w561
                shift-left: w560 -> [w582]
                stop <- w585 continue-if-true
                w571 = ""
                n206 = call <vilib>:"Read File+ (string).vi"("count"=0, "line mode (characters:F)"=TRUE, "error in (no error)"=w582, "refnum"=w589) -> ("error out"=w575:errorcluster, "string"=w584:string, "dup refnum"=w583:refnum<file>, "EOF?"=w587:bool)  [unwired: 3 in, 1 out]
                n207 = Unbundle By Name(w575) -> ("status"=w586:bool)
                n208 = Search/Split String(string=w584, search string/char (-)="%" ("search char (-)")) -> (substring before match=w579:string, match + rest of string=w590:string)  [unwired: 1 in, 1 out]
                n209 = Not Or(1:w587, 2:w586) -> (0:w585:bool)
                n210 = String Subset(string=w590, offset (0)=1) -> (substring=w569:string)  [unwired: 1 in]
                n211 = Search and Replace String(input string=w569, search string="\r", replace string=w571) -> (result string=w570:string)  [unwired: 5 in, 3 out]
                n212 = Search and Replace String(input string=w570, search string="\n", replace string=w571) -> (result string=w568:string)  [unwired: 5 in, 3 out]
                n213 = for {
                  N: w576 -> [_]
                  tunnel: w580 -> [w601] mode=indexing
                  tunnel: w579 -> [w596]
                  shift-right: [w597] -> w577
                  shift-left: w578 -> [w598]
                  tunnel: w568 -> [w595]
                  shift-right: [w593] -> w574
                  shift-left: w575 -> [w594]
                  i -> [w599]
                  n214 = Match Pattern(string=w601, regular expression=w596) -> (offset past match=w602:i32)  [unwired: 1 in, 3 out]
                  n215 = Increment(x=w602) -> (x+1=w603:i32)
                  n216 = Greater Than 0?(x=w603) -> (x > 0?=w600:bool)
                  n217 = case shown="True" w600 {
                    tunnel: w599 -> [_ w611]
                    tunnel: w595 -> [_ w610]
                    tunnel: w598 -> [w605 w609]
                    tunnel: [w605 w608] -> w597
                    tunnel: w594 -> [w604 w607]
                    tunnel: [w604 w606] -> w593
                    frame False {
                    }
                    frame True {
                      n218 = case shown="0, Default" w611 {
                        tunnel: w610 -> [w612 w616 w621 w627 w633 w639 w643 w650 w656 w660 w665 w674 w679 w690 w696 w700]
                        tunnel: w609 -> [w614 w618 w622 w629 w635 w641 w646 w647 w653 w661 w666 w677 w682 w692 w695 w703]
                        tunnel: [w615 w619 w623 w628 w634 w640 w645 w648 w654 w662 w667 w676 w681 w691 w693 w701] -> w608
                        tunnel: w607 -> [w613 w617 w620 w624 w630 w636 w644 w649 w655 w663 w668 w669 w678 w689 w694 w702]
                        tunnel: [w613 w617 w620 w624 w630 w636 w644 w649 w655 w663 w668 w669 w678 w689 w694 w702] -> w606
                        frame 0, Default {
                          n219 = Bundle By Name(cluster=w614, "Bias Supply Name"=w612) -> (w615:T5)
                        }
                        frame 1 {
                          n220 = Bundle By Name(cluster=w618, "SMU Name"=w616) -> (w619:T5)
                        }
                        frame 2 {
                          n221 = Bundle By Name(cluster=w622, "LCR Name"=w621) -> (w623:T5)
                        }
                        frame 3 {
                          n222 = Scan Value(string=w627, format string="%.1f") -> (value=w626:dbl)  [unwired: 1 in, 1 out]
                          n223 = Bundle By Name(cluster=w629, "Bias Voltage [V]"=w626) -> (w628:T5)
                        }
                        frame 4 {
                          n224 = Scan Value(string=w633, format string="%.1f") -> (value=w632:dbl)  [unwired: 1 in, 1 out]
                          n225 = Bundle By Name(cluster=w635, "Base Voltage [V]"=w632) -> (w634:T5)
                        }
                        frame 5 {
                          n226 = Scan Value(string=w639, format string="%.1f") -> (value=w638:dbl)  [unwired: 1 in, 1 out]
                          n227 = Bundle By Name(cluster=w641, "Base Ramp Step [V]"=w638) -> (w640:T5)
                        }
                        frame 6 {
                          n228 = Decimal String To Number(string=w643) -> (number=w642:i32)  [unwired: 2 in, 1 out]
                          n229 = Bundle By Name(cluster=w646, "Base Ramp Interval [ms]"=w642) -> (w645:T5)
                        }
                        frame 7 {
                          n230 = Scan Value(string=w650, format string="%.1f") -> (value=w652:dbl)  [unwired: 1 in, 1 out]
                          n231 = Bundle By Name(cluster=w647, "High Voltage [V]"=w652) -> (w648:T5)
                        }
                        frame 8 {
                          n232 = Scan Value(string=w656, format string="%.1f") -> (value=w658:dbl)  [unwired: 1 in, 1 out]
                          n233 = Bundle By Name(cluster=w653, "High Ramp Step [V]"=w658) -> (w654:T5)
                        }
                        frame 9 {
                          n234 = Decimal String To Number(string=w660) -> (number=w659:i32)  [unwired: 2 in, 1 out]
                          n235 = Bundle By Name(cluster=w661, "High Ramp Interval [ms]"=w659) -> (w662:T5)
                        }
                        frame 10 {
                          n236 = Decimal String To Number(string=w665) -> (number=w664:i32)  [unwired: 2 in, 1 out]
                          n237 = Bundle By Name(cluster=w666, "AC frequency [Hz]"=w664) -> (w667:T5)
                        }
                        frame 11 {
                          w673 = u16 0 items=["serial", "parallel"] ("RC Configuration")
                          w672 = u16 1 items=["serial", "parallel"] ("RC Configuration")
                          n238 = Equal?(x=w674, y="serial") -> (x = y?=w671:bool)
                          n239 = Select(t=w673, s=w671, f=w672) -> (s? t:f=w670:u16)
                          n240 = Bundle By Name(cluster=w677, "RC Configuration"=w670) -> (w676:T5)
                        }
                        frame 12 {
                          n241 = Scan Value(string=w679, format string="%.1f") -> (value=w680:dbl)  [unwired: 1 in, 1 out]
                          n242 = Bundle By Name(cluster=w682, "AC amplitude [V]"=w680) -> (w681:T5)
                        }
                        frame 13 {
                          n243 = Equal?(x=w690, y="Arduino") -> (x = y?=w687:bool)
                          n244 = Select(t=enum16{"Read Arduino", "Enter manually"}."Read Arduino" ("Temperature Readout"), s=w687, f=enum16{"Read Arduino", "Enter manually"}."Enter manually" ("Temperature Readout")) -> (s? t:f=w684:enum16{"Read Arduino", "Enter manually"})
                          n245 = Bundle By Name(cluster=w692, "Temperature Readout"=w684) -> (w691:T5)
                        }
                        frame 14 {
                          n246 = Scan Value(string=w696, format string="%.1f") -> (value=w697:dbl)  [unwired: 1 in, 1 out]
                          n247 = Bundle By Name(cluster=w695, "Fraction of good strips [%]"=w697) -> (w693:T5)
                        }
                        frame 15 {
                          n248 = Decimal String To Number(string=w700) -> (number=w699:i32)  [unwired: 2 in, 1 out]
                          n249 = Bundle By Name(cluster=w703, "Probe Card Channels"=w699) -> (w701:T5)
                        }
                      }
                    }
                  }
                }
              }
              n250 = call <vilib>:"Close File+.vi"("error in (no error)"=w561, "refnum"=w562) -> ()  [unwired: 3 in, 3 out]
            }
            frame Error {
              n251 = One Button Dialog(message="Can't open definitions file!") -> ()  [unwired: 1 in, 1 out]
            }
          }
          n252 = global write "QC_MeasurementSetup.vi" "Striptest Measurement Parameters"(w552) -> ()
        }
      }
    }
  }
